vi "Main.vi"() -> ()   [LabVIEW 2023]
panel:
  out "Result":dbl
  in  "Divide":bool
  in  "Multiply":bool
  in  "Subtract":bool
  in  "Add":bool
  in  "Operand 2":dbl
  in  "Operand 1":dbl
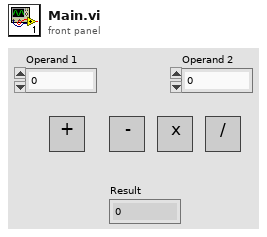
[diagram p1: front panel]
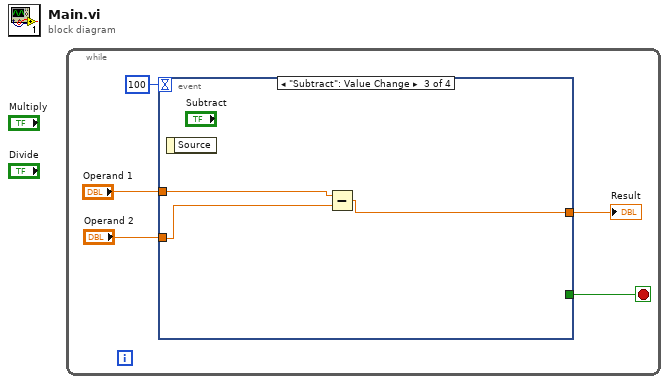
[diagram p0: block diagram]
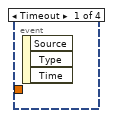
[diagram p2: hidden frame]
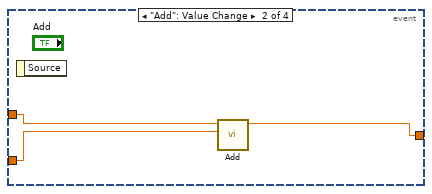
[diagram p3: hidden frame]
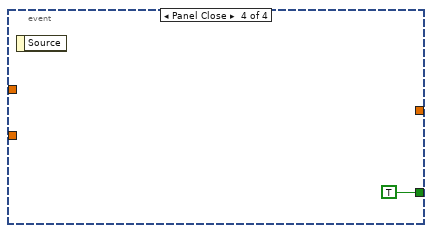
[diagram p4: hidden frame]
diagram:
  n1 = while {
    stop <- w1 stop-if-true
    n2 = event shown="[2] \"Subtract\": Value Change" {
      selector: _ -> [_ _ _ _]
      dyn-events: _ -> [_ _ _ _]
      timeout: 100 -> [_ _ _ _]
      tunnel: "Operand 1" -> [_ w8 w11 _]
      tunnel: "Operand 2" -> [_ w7 w10 _]
      tunnel: [_ w6 w9 _] -> w2
      tunnel: [_ _ _ TRUE] -> w1
      event Timeout {
        n3 = event-data() -> ()  [unwired: 1 in, 3 out]
      }
      event "Add": Value Change {
        n4 = event-data() -> ()  [unwired: 1 in, 1 out]
        n5 = call "Add.vi"("Operand in"=w7, "Operand 1"=w8) -> ("Numeric"=w6:dbl)  [unwired: 9 in]
      }
      event "Subtract": Value Change {
        n6 = event-data() -> ()  [unwired: 1 in, 1 out]
        n7 = Subtract(x=w11, y=w10) -> (x-y=w9:dbl)
      }
      event Panel Close {
        n8 = event-data() -> ()  [unwired: 1 in, 1 out]
      }
    }
    "Result" <- w2
  }
